vi "DOS cmd.vi"(8 "错误输入（无错误）":errorcluster, 11 "批处理文件路径":path) -> (0 "error out":errorcluster caption="错误输出")   [LabVIEW 2016, in "update.lvlib"]
uses:
  update.lvlib
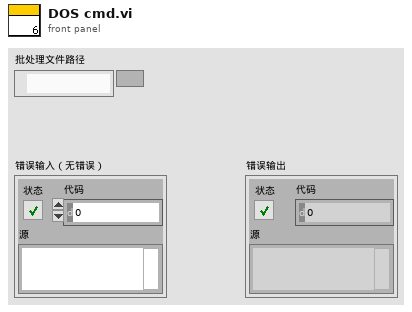
[diagram p1: front panel]
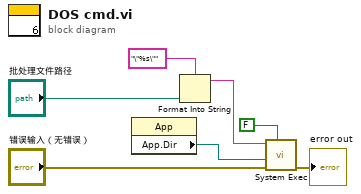
[diagram p0: block diagram]
diagram:
  n1 = property class="App"() -> ("App.Dir"=w4:path)  [unwired: 2 in, 2 out]
  n2 = Format Into String(format string="\"%s\"" ("格式字符串"), "批处理文件路径") -> (resulting string=w1:string)  [unwired: 2 in, 1 out]
  n3 = call <vilib>:"System Exec.vi"("wait until completion? (T)"=FALSE, "error in (no error)"="错误输入（无错误）", "working directory"=w4, "command line"=w1) -> ("error out"=→"error out":errorcluster)  [unwired: 4 in, 3 out]
